vi "Func Input.vi"(7 "Actor":refnum<class "Actor Layer.lvclass">, 11 "Actor":T1) -> (3 "Actor":T1)   [LabVIEW 2020, in "jettl.lvlib"]
uses:
  jettl.lvlib
  Actor Layer/Actor Layer.lvclass
  Msg/Msg.lvclass
  Origin.ctl
  Lifecycle.ctl
  Msg Attribs.ctl
  Msg.ctl
  Post Setup.ctl
  Pre Setup.ctl
  Msg Set.ctl
  Layer Type.ctl
  Layer Attribs.ctl
  Layer Map.ctl
  Implemented Map.ctl
  Actor Attribs.ctl
  Children.ctl
  Actor.ctl
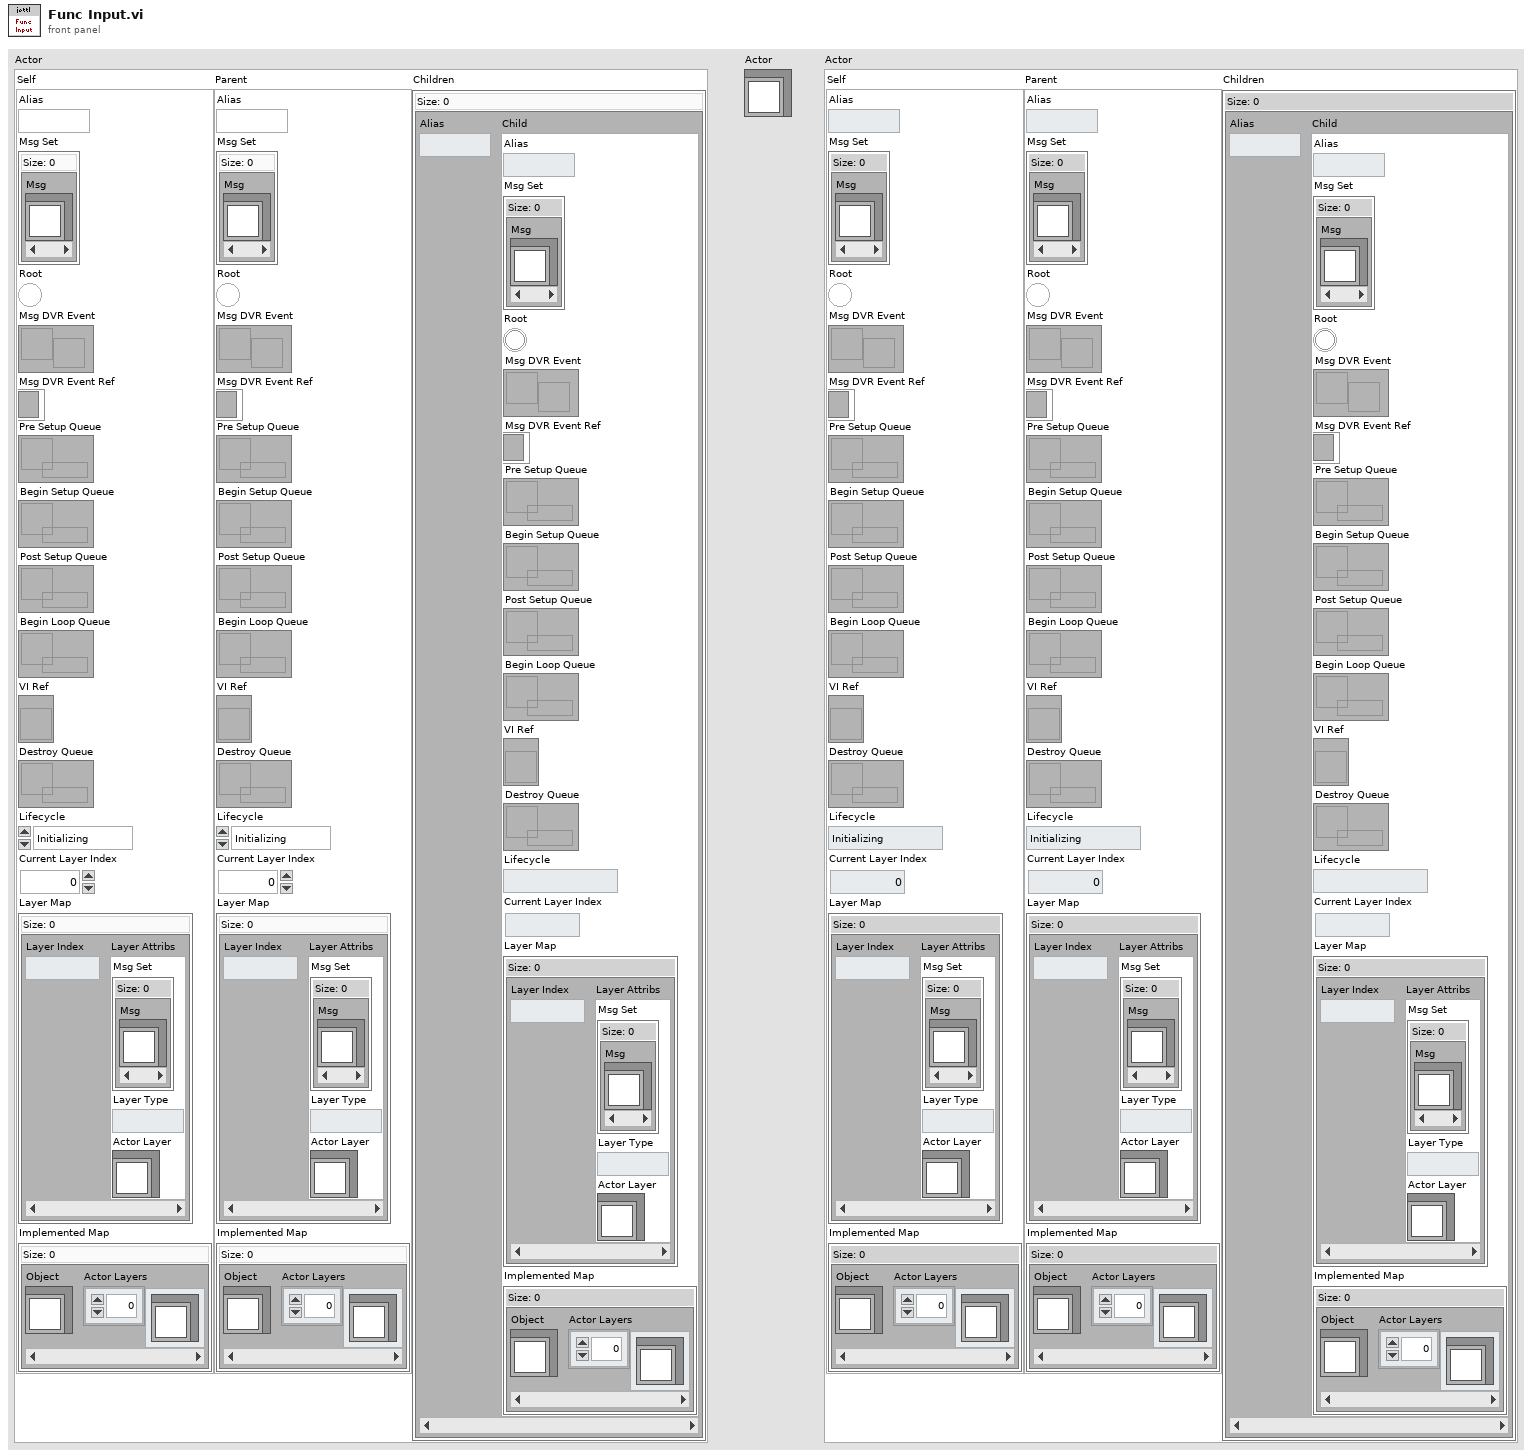
[diagram p1: front panel]
types:
  T1 = typedef "jettl.lvlib/Actor.ctl" = cluster{"Self":T2, "Parent":T2, "Children":T9}
  T2 = typedef "jettl.lvlib/Actor Attribs.ctl" = cluster{"Alias":string, "Msg Set":T3, "Root":bool, "Msg DVR Event":refnum<user-event>, "Msg DVR Event Ref":refnum<event-registration>, "Pre Setup Queue":refnum<queue>, "Begin Setup Queue":refnum<queue>, "Post Setup Queue":refnum<queue>, "Begin Loop Queue":refnum<queue>, "VI Ref":refnum<vi>, "Destroy Queue":refnum<queue>, "Lifecycle":T4, "Current Layer Index":i32, "Layer Map":T5, "Implemented Map":T8}
  T3 = typedef "jettl.lvlib/Msg Set.ctl" = set{refnum<class "Msg.lvclass">}
  T4 = typedef "jettl.lvlib/Lifecycle.ctl" = enum16{"Initializing", "Setting Up", "Starting", "Running", "Stopping", "Tearing Down", "Terminated"}
  T5 = typedef "jettl.lvlib/Layer Map.ctl" = map{i32, T6}
  T6 = typedef "jettl.lvlib/Layer Attribs.ctl" = cluster{"Msg Set":T3, "Layer Type":T7, "Actor Layer":refnum<class "Actor Layer.lvclass">}
  T7 = typedef "jettl.lvlib/Layer Type.ctl" = enum16{"Base", "InnerGlobal", "InnerLocal", "Outer"}
  T8 = typedef "jettl.lvlib/Implemented Map.ctl" = map{refnum<class>, refnum<class "Actor Layer.lvclass">[]}
  T9 = typedef "jettl.lvlib/Children.ctl" = map{string, T2}
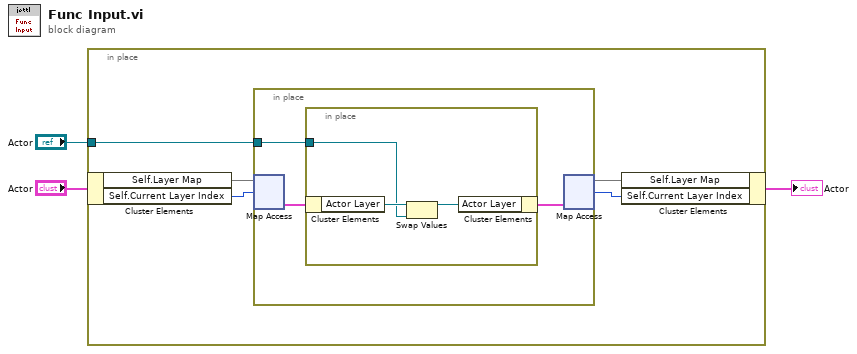
[diagram p0: block diagram]
diagram:
  n1 = in-place {
    in-place-border: "Actor" -> [w6]
    n2 = in-place-cluster #1("Actor") -> ("Self.Layer Map"=w8:T5, "Self.Current Layer Index"=w5:i32)
    n3 = in-place {
      in-place-border: w6 -> [w9]
      n4 = in-place-map #2(w8, w5) -> (w11:T6)  [unwired: 1 in, 1 out]
      n5 = in-place {
        in-place-border: w9 -> [w13]
        n6 = in-place-cluster #3(w11) -> ("Actor Layer"=w14:refnum<class "Actor Layer.lvclass">)
        n7 = Swap Values(12:w14, 14:w13) -> (1:w12:refnum<class "Actor Layer.lvclass">)  [unwired: 1 in, 1 out]
        n8 = in-place-cluster #3("Actor Layer"=w12) -> (w10:T6)
      }
      n9 = in-place-map #2(w10) -> (w7:T5, w4:i32)  [unwired: 1 in, 1 out]
    }
    n10 = in-place-cluster #1("Self.Layer Map"=w7, "Self.Current Layer Index"=w4) -> (→"Actor":T1)
  }
